vi "dataUserOut.vi"(8 "error in (no error) 2":errorcluster) -> (0 "error out 2":errorcluster, 3 "Data":string[][](array[string]))   [LabVIEW 2014]
uses:
  <vilib>/addons/database/Connection.llb/DB Tools Open Connec (String).vi
  <vilib>/addons/database/Connection.llb/Conn Execute.vi
  <vilib>/addons/database/Recordset.llb/Rec Fetch Recordset Data (R).vi
  <vilib>/addons/database/Recordset.llb/Rec Destroy - Connection.vi
  <vilib>/addons/database/_DB Variant To Data/Database Variant To Data.xnode
  <vilib>/addons/database/NI_Database_API.lvlib
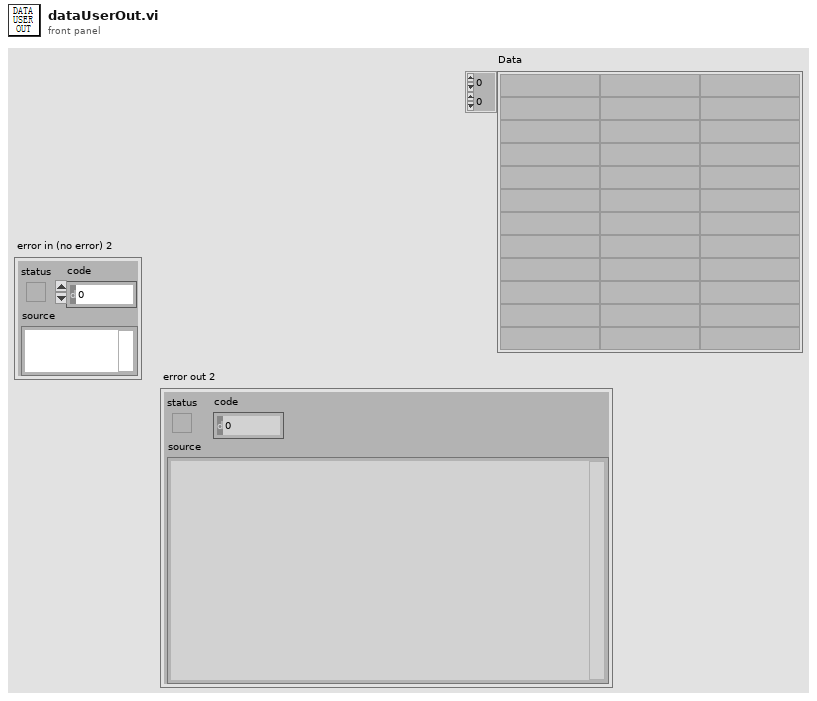
[diagram p1: front panel]
types:
  T1 = typedef "NI_Database_API.lvlib/Conn ObjectReference.ctl" = refnum<k1>
  T2 = typedef "NI_Database_API.lvlib/Rec ObjectReference.ctl" = refnum<k1>
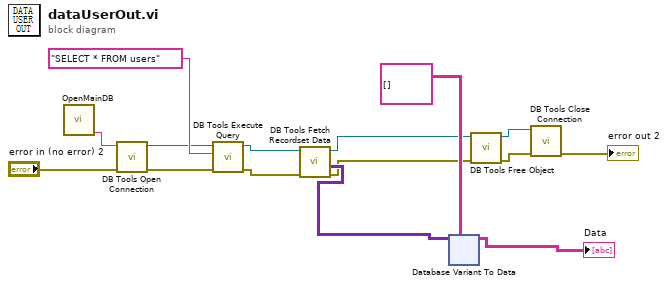
[diagram p0: block diagram]
diagram:
  n1 = call "OpenMainDB.vi"() -> ("头信息"=w2:string)  [unwired: 11 in]
  n2 = call-poly <vilib>:"DB Tools Open Connection.vi"("error in (no error)"="error in (no error) 2", "connection information"=w2) -> ("error out"=w6:errorcluster, "connection reference"=w5:T1)  [unwired: 6 in]
  n3 = call-poly <vilib>:"DB Tools Execute Query.vi"("error in (no error)"=w6, "SQL query"="SELECT * FROM users", "connection reference"=w5) -> ("error out"=w7:errorcluster, "recordset reference"=w4:T2)  [unwired: 5 in]
  n4 = call-poly <vilib>:"DB Tools Fetch Recordset Data.vi"("error in (no error)"=w7, "recordset reference"=w4) -> ("error out"=w10:errorcluster, "recordset data"=w15:variant[][], "recordset reference out"=w9:T2)  [unwired: 3 in]
  n5 = xnode "Database Variant To Data"("database variant"=w15, "type"=string[][] []) -> ("data"=→"Data":string[][])  [unwired: 1 in, 1 out]
  n6 = call-poly <vilib>:"DB Tools Free Object.vi"("error in (no error)"=w10, "recordset reference"=w9) -> ("error out"=w12:errorcluster, "connection reference"=w11:T1)  [unwired: 8 in]
  n7 = call <vilib>:"DB Tools Close Connection.vi"("error in (no error)"=w12, "connection reference"=w11) -> ("error out"=→"error out 2":errorcluster)  [unwired: 5 in]
